vi "Error Constant Template.vi"   [LabVIEW 2016]
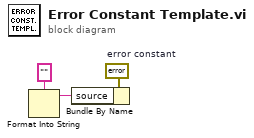
[diagram p0: block diagram]
diagram:
  w3 = errorcluster {"status"=TRUE, "code"=0, "source"=""}  # error constant
  n1 = Format Into String(format string="") -> (resulting string=w2:string)  [unwired: 3 in, 1 out]
  n2 = Bundle By Name(cluster=w3, "source"=w2) -> ()  [unwired: 1 out]
